vi "_Process Start Run.vi"(7 "Ready":bool, 8 "Error In":errorcluster, 9 "binary string":string, 11 "Command":T1) -> (0 "Error Out":errorcluster, 2 "RunMode":i32, 3 "Running":bool)   [LabVIEW 2015]
uses:
  Type/_RT Command.ctl
  Type/_RT Parameter.ctl
  Type/_RT Active Ch.ctl
  Type/_RT Expt.ctl
  Type/_Run Mode.ctl
  Type/_RT Mass Range.ctl
  Type/_RT Res Type.ctl
  _RT Global.vi
  <vilib>/Utility/error.llb/Error Cluster From Error Code.vi
  <vilib>/rvi/errors/niLvFpgaAdjustHostInterfaceError.vi
  <vilib>/rvi/interface/nirviReadWriteControl/nirviReadWriteControl.xnode
  Type/FPGA Typedef.ctl
  FPGA Bitfiles/FPGA9607.lvbitx
  NiFpgaLv.dll
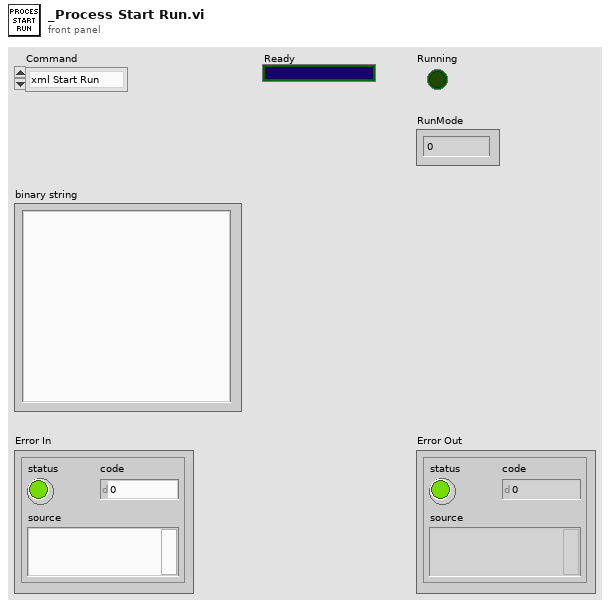
[diagram p1: front panel]
types:
  T1 = typedef "_RT Command.ctl" = enum16{"xml Start Run", "xml Start Actual Run", "xml Stop Run", "xml Runtime Update", "xml Get Status", "xml Get Table", "xml Set Table", "xml Get Configuration", "xml System Status", "xml Set LC Input Logic", "xml Get Data", "xml Get Info", "Start", "StartActualRun", "Stop", "Runtime Update", "Get Data", "Get Info", "Get Status", "Get Param", "Get Config", "Get Table", "Read ADC", "Set Oscillator", "Update Config", "Update Table", "Set All Pol", "Set Pol and DC", "Set Max Mass", "Toggle RP", "Toggle EL", "Set PIC", "Initialize Turbo", "Send Turbo Comm", "Close Turbo", "P1", "P2", "P3", "Send Serial", "Set LC Out", "Get LC In", "Read VAC", "Test Table", "Toggle Power", "Get Startup", "Set Startup", "Get ADC Table", "Set ADC Table", "Get Brief Status", "Get Detail Status", "Auxiliary Update", "Set CC Logics", "Set CC Input Logics", "Ignore Error", "invalid"}
  T2 = typedef "Semaphore RefNum" = refnum<k1>
  T3 = typedef "_RT Instrument State.ctl" = enum16{"Initializing", "Mass Spectrometer is Off", "Starting Up", "Turning Power Off", "Going to Standby", "Roughing Pump Ready", "Turning Turbo Off", "Turbo Startup", "Turbopump Ready", "Checking Vacuum", "Going to Ready", "Ready", "Running", "Source Standby", "Lost Communication", "Shutting Down", "Fault", "24V Standby", "Go to 24V Standby", "Turbopump Ready-Waiting"}
  T4 = typedef "_RT Parameter.ctl" = cluster{"RunMode":i32, "Initial Ch":T5[], "Sync":u8, "Expt":T6[], "EqTime(mS)":i32}
  T5 = typedef "_RT Active Ch.ctl" = cluster{"Start":i32, "Step":i32, "ChID":i32}
  T6 = typedef "_RT Expt.ctl" = cluster{"StartT(mS)":i32, "#Cycles":i32, "Scan Type":T7, "PauseT(uS)":i32, "Polarity":u8, "DelayT(mS)":i32, "Active Ch":T5[], "Mass Range":T8[]}
  T7 = typedef "_Run Mode.ctl" = enum16{"MRM (Q1/Q2)", "Q1 Scan", "Q1 SRM", "Q2 Scan", "Q2 SRM", "Product Scan", "Precursor Scan", "Neutral Loss", "Neutral Gain"}
  T8 = typedef "_RT Mass Range.ctl" = cluster{"Steps":i32, "Dwell(uS)":i32, "Resolution Type":T9, "Ramping Ch":T5[]}
  T9 = typedef "_RT Res Type.ctl" = u16
  T10 = typedef "_XML Lens.ctl" = cluster{"Value":dbl, "ChID":u8}
  T11 = typedef "_Server Method.ctl" = cluster{"RunMode":i32, "Sync":u8, "Expt":T12[], "EqTime(mS)":i32, "TuneParam":T5[]}
  T12 = typedef "_XML Expt.ctl" = cluster{"StartT(mS)":i32, "#Cycles":i32, "PauseT(uS)":i32, "ScanType":i32, "Polarity":u8, "FixedMass":dbl, "DelayT(mS)":i32, "Active Ch":T10[], "Mass Range":T13[]}
  T13 = typedef "_Mass Range Property.ctl" = cluster{"Start":dbl, "Stop":dbl, "Step Size":dbl, "Steps":i32, "Dwell":dbl, "Parameters":T14[], "Res":T9}
  T14 = typedef "_Mass Range Parameters.ctl" = cluster{"Name":string, "Ch#":u8, "StartV":dbl, "StopV":dbl, "StepV":dbl, "Index":u8}
  T15 = typedef "FPGA Typedef.ctl" = refnum<k20>
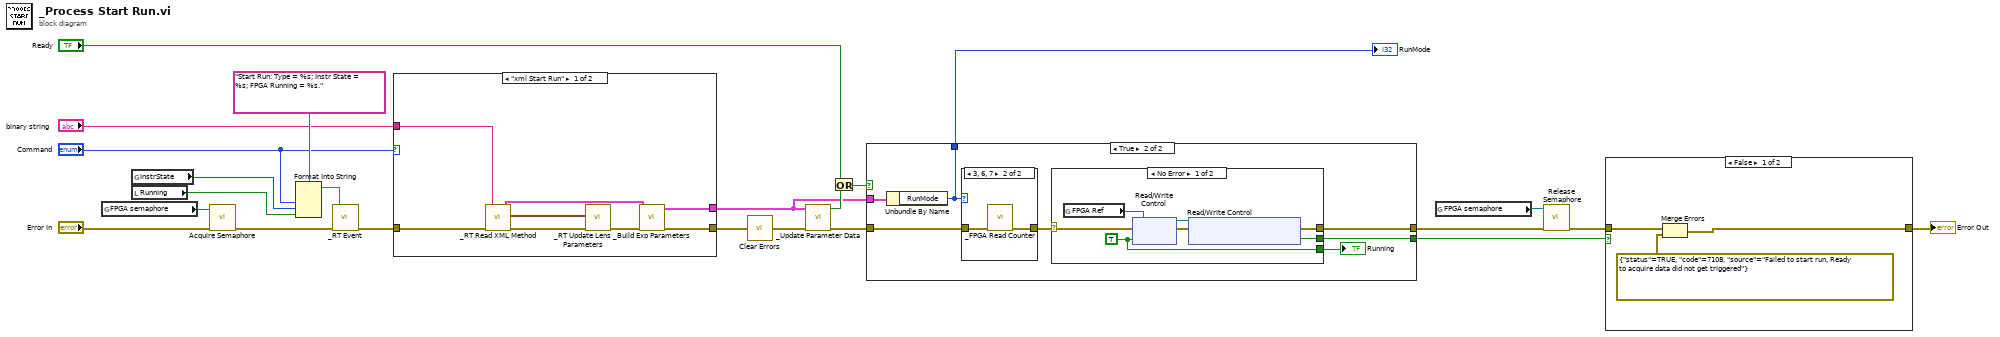
[diagram p0: block diagram]
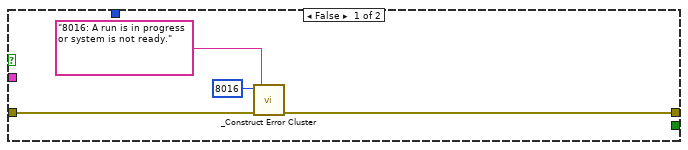
[diagram p3: hidden frame]
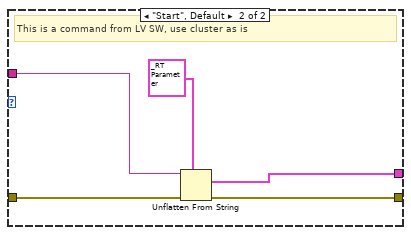
[diagram p6: hidden frame]
diagram:
  n1 = global read "_RT Global.vi" "FPGA semaphore"() -> (w6:T2)
  n2 = global read "_RT Global.vi" "InstrState"() -> (w19:T3)
  n3 = local read "Running"() -> (w23:bool)
  n4 = call <vilib>:"Acquire Semaphore.vi"("error in (no error)"="Error In", "semaphore"=w6) -> ("error out"=w7:errorcluster)  [unwired: 3 in, 2 out]
  n5 = Format Into String(format string="Start Run: Type = %s; Instr State = %s; FPGA Running = %s.", "Command", w19, w23) -> (resulting string=w21:string)  [unwired: 2 in, 1 out]
  n6 = call "_RT Event.vi"("error in (no error)"=w7, "Event"=w21) -> ("error out"=w20:errorcluster)  [unwired: 1 in, 4 out]
  n7 = case shown="\"xml Start Run\"" "Command" {
    tunnel: [w27 w35] -> w14
    tunnel: w20 -> [w31 w36]
    tunnel: [w25 w32] -> w13
    tunnel: "binary string" -> [w24 w34]
    frame "xml Start Run" {
      n8 = call "_RT Read XML Method.vi"("error in"=w31, "XML String"=w24) -> ("error out"=w30:errorcluster, "Lens"=w29:T10[], "Server Method"=w26:T11)  [unwired: 3 in]
      n9 = call "_RT Update Lens Parameters.vi"("error in"=w30, "Lens"=w29) -> ("error out"=w28:errorcluster)  [unwired: 9 in]
      n10 = call "_Build Exp Parameters.vi"("error in (no error)"=w28, "Server Method"=w26) -> ("error out"=w27:errorcluster, "Exp Parameters"=w25:T4)  [unwired: 8 in]
    }
    frame "Start", Default {
      # "This is a command from LV SW, use cluster as is"
      n11 = Unflatten From String(type=T4 {"RunMode"=3, "Initial Ch"=[], "Sync"=0, "Expt"=[{"StartT(mS)"=0, "#Cycles"=200, "Scan Type"=enum."Q1 Scan", "PauseT(uS)"=0, "Polarity"=0, "DelayT(mS)"=0, "Active Ch"=[], "Mass Range"=[{"Steps"=2000, "Dwell(uS)"=100, "Resolution Type"=0, "Ramping Ch"=[{"Start"=20000, "Step"=81920, "ChID"=1}, {"Start"=20000, "Step"=81920, "ChID"=4}, {"Start"=20000, "Step"=81920, "ChID"=7}, {"Start"=20000, "Step"=81920, "ChID"=2}, {"Start"=20000, "Step"=81920, "ChID"=5}, {"Start"=20000, "Step"=81920, "ChID"=9}]}]}], "EqTime(mS)"=0} ("Parameter"), binary string=w34, error in (no error)=w36) -> (value=w32:T4, error out=w35:errorcluster)  [unwired: 3 out]
    }
  }
  n12 = call <vilib>:"Clear Errors.vi"("error in (no error)"=w14) -> ("error out"=w9:errorcluster)  [unwired: 5 in, 1 out]
  n13 = call "_Update Parameter Data.vi"("error in"=w9, "Parameter"=w13) -> ("error out"=w17:errorcluster, "RF Only"=w16:bool)  [unwired: 1 in, 3 out]
  n14 = Or(x="Ready", y=w16) -> (x .or. y?=w15:bool)
  n15 = case shown="True" w15 {
    tunnel: w13 -> [_ w47]
    tunnel: [w39 w43] -> w5
    tunnel: w17 -> [w37 w44]
    tunnel: [_ w42] -> w10
    tunnel: [_ w41] -> w3
    frame False {
      n16 = call "_Construct Error Cluster.vi"("error in"=w37, "reason"="8016: A run is in progress or system is not ready.", "errorCode"=8016) -> ("error out"=w39:errorcluster)  [unwired: 1 in, 3 out]
    }
    frame True {
      n17 = Unbundle By Name(w47) -> ("RunMode"=w42:i32)
      n18 = case shown="3, 6, 7" w42 {
        tunnel: w44 -> [w48 w50]
        tunnel: [w48 w49] -> w46
        frame 0, Default {
        }
        frame 3, 6, 7 {
          n19 = call "_FPGA Read Counter.vi"("error in (no error)"=w50) -> ("error out"=w49:errorcluster)  [unwired: 8 in, 2 out]
        }
      }
      n20 = case shown="No Error" w46 {
        selector: w46 -> [w57 w58]
        tunnel: [w52 w58] -> w43
        tunnel: [w55 _] -> w45
        tunnel: [w51 _] -> w41
        frame No Error {
          w55 = TRUE ("Start")
          n21 = global read "_RT Global.vi" "FPGA Ref"() -> (w56:T15)
          n22 = xnode "Read/Write Control"("FPGA VI Reference In"=w56, "error in"=w57, "Start"=w55) -> ("FPGA VI Reference Out"=w54:T15, "error out"=w53:errorcluster)
          n23 = xnode "Read/Write Control"("FPGA VI Reference In"=w54, "error in"=w53) -> ("error out"=w52:errorcluster, "Ready to Acquire Data"=w51:bool)  [unwired: 1 out]
        }
        frame Error {
        }
      }
      "Running" <- w45
    }
  }
  "RunMode" <- w10
  n24 = global read "_RT Global.vi" "FPGA semaphore"() -> (w4:T2)
  n25 = call <vilib>:"Release Semaphore.vi"("error in (no error)"=w5, "semaphore"=w4) -> ("error out"=w2:errorcluster)  [unwired: 4 in, 1 out]
  n26 = case shown="False" w3 {
    tunnel: w2 -> [w61 w62]
    tunnel: [w60 w62] -> w1
    frame False {
      n27 = Merge Errors(w61, errorcluster {"status"=TRUE, "code"=7108, "source"="Failed to start run, Ready to acquire data did not get triggered"} ("error in")) -> (w60:errorcluster)
    }
    frame True {
    }
  }
  "Error Out" <- w1
